vi "DAQmx Create Channel (CI-GPS Timestamp).vi"(0 "task in":refnum<k21>, 1 "gps synchronization method":i32(ring)=10070 items=["IRIG-B"=10070, "PPS"=10080, "None"=10230], 5 "counter":tag, 7 "name to assign":string, 9 "units":i32(ring)=10364 items=["Seconds"=10364, "From Custom Scale"=10065], 11 "error in":errorcluster, 12 "custom scale name":tag) -> (4 "task out":refnum<k21>, 15 "error out":errorcluster)   [LabVIEW 2020]
doc: "Creates a channel that uses a special purpose counter to take a timestamp and synchronizes that counter to a GPS receiver. With the exception of devices that support multi-counter tasks, you can create only one counter input channel at a time with this VI because a task can contain only one counter input channel. To read from multiple counters simultaneously, use a separate task for each counter. Connect the input signals to the default input terminals of the counter unless you select different input terminals."
uses:
  nilvaiu.dll
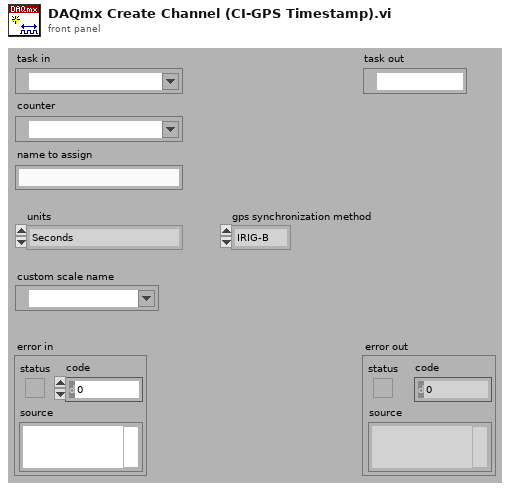
[diagram p1: front panel]
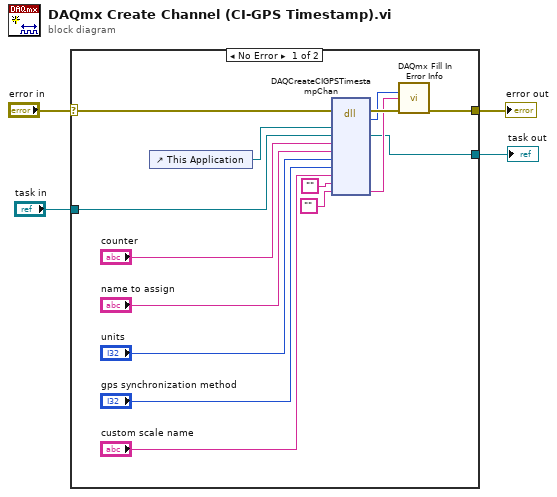
[diagram p0: block diagram]
diagram:
  n1 = case shown="No Error" "error in" {
    selector: "error in" -> [w6 w21]
    tunnel: [w11 w21] -> w4
    tunnel: [w10 w20] -> w3
    tunnel: "task in" -> [w8 w20]
    frame No Error {
      n2 = control-ref of="This Application"() -> (w19:refnum<vi>)
      n3 = dll-call lib="nilvaiu.*" fn="DAQCreateCIGPSTimestampChan"(error in=w6, "lvAppRef"=w19, "refObjPtr"=w8, "counter"="counter", "channelNameIn"="name to assign", "units"="units", "syncMethod"="gps synchronization method", "customScaleName"="custom scale name", "channelNamesOut"="", "extendedErrorInfo"="") -> (error out=w17:errorcluster, "return type"=w16:i32, "refObjPtr"=w10:refnum<k21>, "extendedErrorInfo"=w15:string)  [unwired: 9 in, 1 out]
      n4 = call "DAQmx Fill In Error Info.vi"("status code"=w16, "extended error info"=w15, "error in"=w17) -> ("error out"=w11:errorcluster)  [unwired: 1 in, 11 out]
    }
    frame Error {
    }
  }
  "error out" <- w4
  "task out" <- w3
